vi "weideman64_not_optimized.vi"(6 "N":i32, 9 "imag_in":dbl, 10 "real_in":dbl) -> (2 "imag_out":dbl, 3 "real_out":dbl)   [LabVIEW 2022 SP3]
uses:
  <vilib>/Analysis/2dsp.llb/Real FFT.vi
  <vilib>/Analysis/NI_AALPro.lvlib
panel:
  out "double precision complex":cdb
  out "reversed array":cdb[](array[numeric])
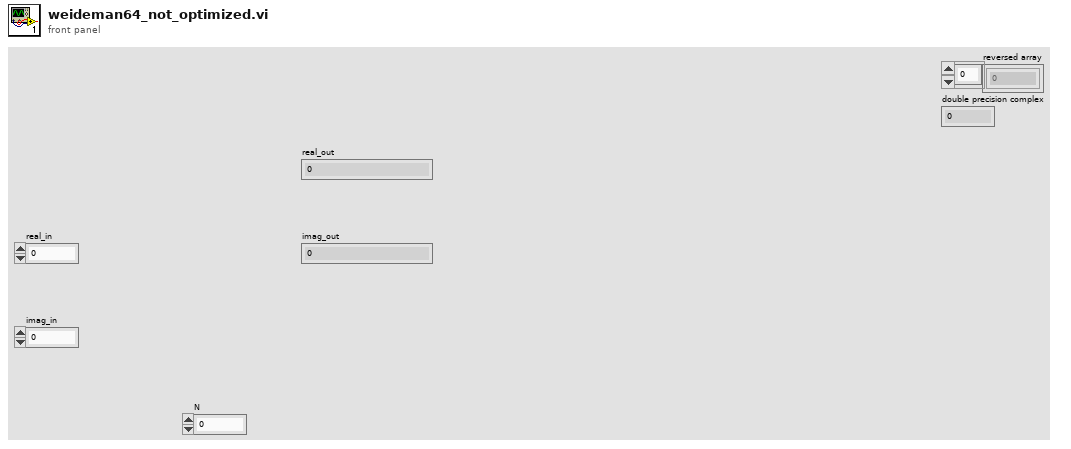
[diagram p1: front panel]
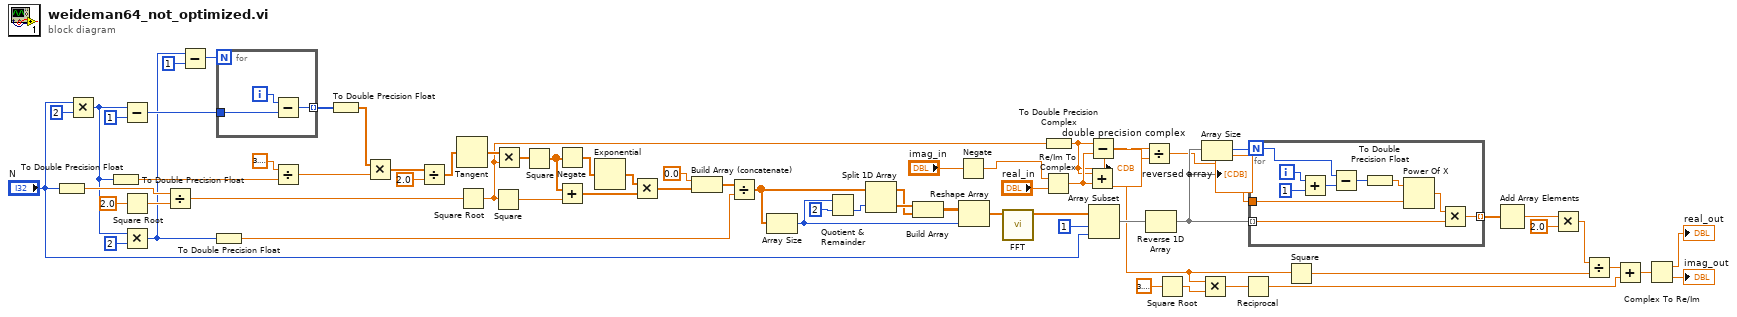
[diagram p0: block diagram]
diagram:
  n1 = To Double Precision Float(number="N") -> (double precision float=w56:dbl)
  n2 = Multiply(x="N", y=2) -> (x*y=w52:i32)
  n3 = To Double Precision Float(number=w52) -> (double precision float=w55:dbl)
  n4 = Subtract(x=w52, y=1 ("x")) -> (x-y=w62:i32)
  n5 = Square Root(x=2.0) -> (sqrt(x)=w61:dbl)
  n6 = Multiply(x=w52, y=2) -> (x*y=w40:i32)
  n7 = Divide(x=w56, y=w61) -> (x/y=w59:dbl)
  n8 = Subtract(x=w40, y=1 ("x")) -> (x-y=w65:i32)
  n9 = To Double Precision Float(number=w40) -> (double precision float=w22:dbl)
  n10 = for {
    N: w65 -> [_]
    tunnel: [w70] -> w58 mode=indexing
    tunnel: w62 -> [w68]
    i -> [w69]
    n11 = Subtract(x=w69, y=w68) -> (x-y=w70:i32)
  }
  n12 = Divide(x=3.141592653589793, y=w55) -> (x/y=w53:dbl)
  n13 = To Double Precision Float(number=w58) -> (double precision float=w57:dbl[])
  n14 = Multiply(x=w57, y=w53) -> (x*y=w51:dbl[])
  n15 = Divide(x=w51, y=2.0 ("x")) -> (x/y=w49:dbl[])
  n16 = Tangent(1:w49) -> (0:w45:dbl[])
  n17 = Square Root(x=w59) -> (sqrt(x)=w2:dbl)
  n18 = Square(x=w2) -> (x^2=w48:dbl)
  n19 = Multiply(x=w45, y=w2) -> (x*y=w44:dbl[])
  n20 = Square(x=w44) -> (x^2=w47:dbl[])
  n21 = Negate(x=w47) -> (-x=w43:dbl[])
  n22 = Add(x=w47, y=w48) -> (x+y=w46:dbl[])
  n23 = Exponential(1:w43) -> (0:w42:dbl[])
  n24 = Multiply(x=w42, y=w46) -> (x*y=w23:dbl[])
  n25 = Build Array (concatenate)(0.0 ("element"), w23) -> (w21:dbl[])
  n26 = Divide(x=w21, y=w22) -> (x/y=w24:dbl[])
  n27 = Array Size(array=w24) -> (size(s)=w34:i32)
  n28 = Quotient & Remainder(x=w34, y=2) -> (floor(x/y)=w38:i32)  [unwired: 1 out]
  n29 = Split 1D Array(array=w24, index=w38) -> (first subarray=w36:dbl[], second subarray=w37:dbl[])
  n30 = Build Array(w37, w36) -> (w35:dbl[][])
  n31 = Negate(x="imag_in") -> (-x=w28:dbl)
  n32 = Reshape Array(w35, w34) -> (w25:dbl[])
  n33 = call-poly <vilib>:"FFT.vi"("X"=w25) -> ("FFT {X}"=w31:cdb[])  [unwired: 9 in, 1 out]
  n34 = Re/Im To Complex(1:"real_in", 2:w28) -> (0:w26:cdb)
  n35 = To Double Precision Complex(1:w2) -> (0:w1:cdb)
  "double precision complex" <- w1
  n36 = Add(x=w1, y=w26) -> (x+y=w4:cdb)
  n37 = Subtract(x=w1, y=w26) -> (x-y=w13:cdb)
  n38 = Array Subset(array=w31, index=1, length="N") -> (w30:cdb[])
  n39 = Divide(x=w4, y=w13) -> (x/y=w3:cdb)
  n40 = Reverse 1D Array(array=w30) -> (reversed array=w19:cdb[])
  "reversed array" <- w19
  n41 = Square Root(x=3.141592653589793) -> (sqrt(x)=w14:dbl)
  n42 = Multiply(x=w13, y=w14) -> (x*y=w7:cdb)
  n43 = Array Size(array=w19) -> (size(s)=w20:i32)
  n44 = Reciprocal(x=w7) -> (1/x=w6:cdb)
  n45 = for {
    N: w20 -> [w80]
    tunnel: w19 -> [w79] mode=indexing
    tunnel: w3 -> [w72]
    tunnel: [w78] -> w18 mode=indexing
    i -> [w76]
    n46 = Add(x=w76, y=1 ("x")) -> (x+y=w75:i32)
    n47 = Subtract(x=w80, y=w75) -> (x-y=w73:i32)
    n48 = To Double Precision Float(number=w73) -> (double precision float=w71:dbl)
    n49 = Power Of X(1:w72, 2:w71) -> (0:w74:cdb)
    n50 = Multiply(x=w74, y=w79) -> (x*y=w78:cdb)
  }
  n51 = Square(x=w13) -> (x^2=w9:cdb)
  n52 = Add Array Elements(numeric array=w18) -> (sum=w12:cdb)
  n53 = Multiply(x=w12, y=2.0 ("x")) -> (x*y=w10:cdb)
  n54 = Divide(x=w10, y=w9) -> (x/y=w8:cdb)
  n55 = Add(x=w8, y=w6) -> (x+y=w5:cdb)
  n56 = Complex To Re/Im(x + iy=w5) -> (x=→"real_out":dbl, y=→"imag_out":dbl)
